vi "Output_Trav_Pos_low.vi"(4 "Positions to Output":T1) -> (1 "error out":errorcluster)   [LabVIEW 2011]
uses:
  Controls/Positions.ctl
  Globals/Trav_pos_global.vi
  <userlib>/LV-Link3/PolySubVIs/DtCreateAoutChan.vi
  Route mapping/Route_mapping_global.vi
  <userlib>/LV-Link3/PolySubVIs/DtOLWriteSingle.vi
  <userlib>/LV-Link3/PolySubVIs/DtOLWriteMultiple2D.vi
panel:
  out "X, Y, Z":dbl[](array[numeric])
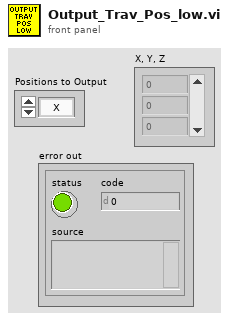
[diagram p1: front panel]
types:
  T1 = typedef "Positions.ctl" = enum16{"X", "Y", "Z", "XY", "XZ", "YZ", "XYZ"}
  T2 = typedef "Box_size.ctl" = cluster{"Max":dbl, "Min":dbl}[]
  T3 = enum32{"Bad", "Idle", "Run top level", "Running"}
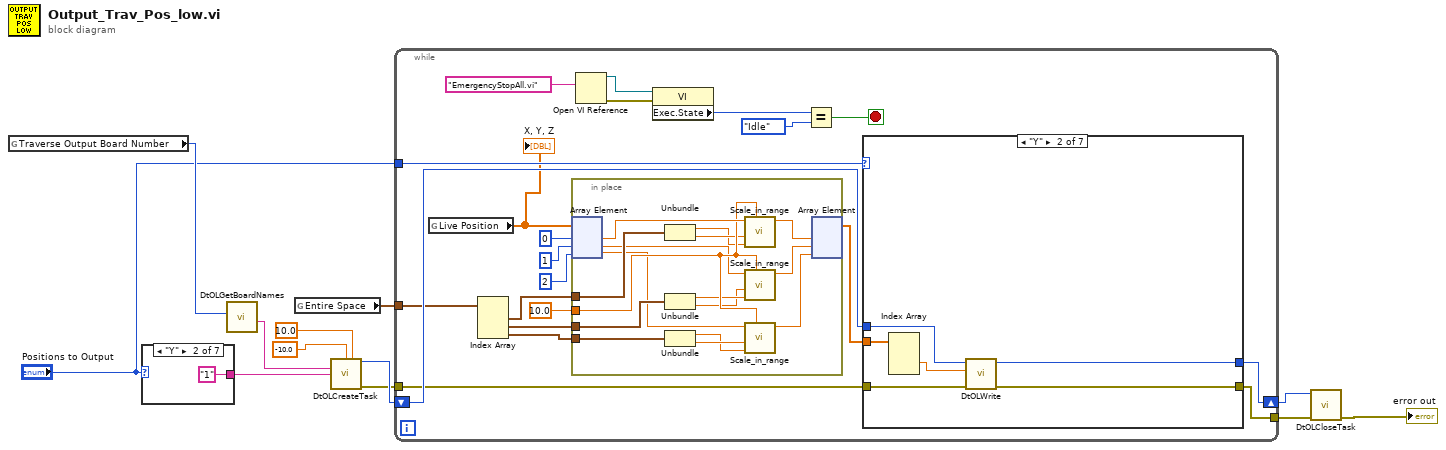
[diagram p0: block diagram]
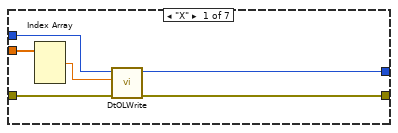
[diagram p2: hidden frame]
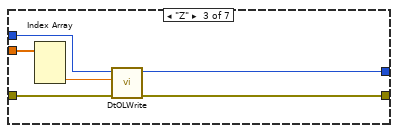
[diagram p3: hidden frame]
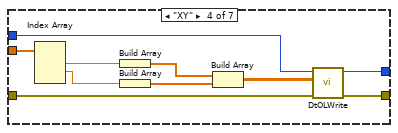
[diagram p4: hidden frame]
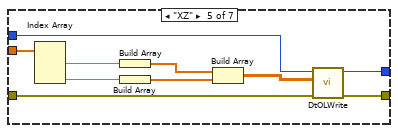
[diagram p5: hidden frame]
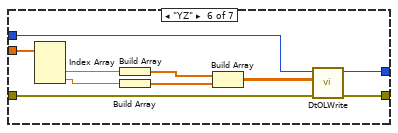
[diagram p6: hidden frame]
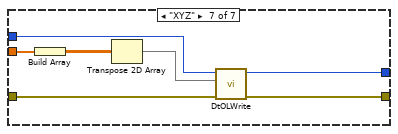
[diagram p7: hidden frame]
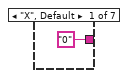
[diagram p8: hidden frame]
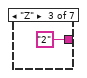
[diagram p9: hidden frame]
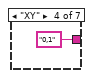
[diagram p10: hidden frame]
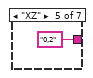
[diagram p11: hidden frame]
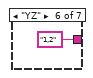
[diagram p12: hidden frame]
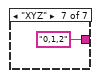
[diagram p13: hidden frame]
diagram:
  n1 = global read "Trav_pos_global.vi" "Traverse Output Board Number"() -> (w6:u32)
  n2 = case shown="\"Y\"" "Positions to Output" {
    tunnel: ["0" ("Channel") "1" ("Channel") "2" ("Channel") "0,1" ("Channel") "0,2" ("Channel") "1,2" ("Channel") "0,1,2" ("Channel")] -> w8
    frame "X", Default {
    }
    frame "Y" {
    }
    frame "Z" {
    }
    frame "XY" {
    }
    frame "XZ" {
    }
    frame "YZ" {
    }
    frame "XYZ" {
    }
  }
  n3 = call <userlib>:"DtOLGetBoardNames.vi"("Select Board"=w6) -> ("Board Name"=w9:string)  [unwired: 8 in, 2 out]
  n4 = global read "Route_mapping_global.vi" "Entire Space"() -> (w5:T2)
  n5 = call-poly <userlib>:"DtOLCreateTask.vi"("Range Min"=-10.0, "Range Max"=10.0, "Board Name"=w9, "Channel"=w8) -> ("Task out"=w10:i32, "error out"=w7:errorcluster)  [unwired: 9 in, 1 out]
  n6 = while {
    shift-right: [w40] -> w1
    shift-left: w10 -> [w39]
    tunnel: "Positions to Output" -> [w38]
    tunnel: w7 -> [w31]
    tunnel: [w30] -> w3
    tunnel: w5 -> [w27]
    stop <- w32 stop-if-true
    n7 = global read "Trav_pos_global.vi" "Live Position"() -> (w20:dbl[])
    "X, Y, Z" <- w20
    n8 = Index Array(array=w27) -> (element #1=w26:cluster{"Max":dbl, "Min":dbl}, element #2=w25:cluster{"Max":dbl, "Min":dbl}, element #3=w24:cluster{"Max":dbl, "Min":dbl})  [unwired: 3 in]
    n9 = in-place {
      in-place-border: 10.0 ("Scale Factor") -> [w55]
      in-place-border: w26 -> [w54]
      in-place-border: w25 -> [w51]
      in-place-border: w24 -> [w50]
      n10 = in-place-array #1(w20, 0, 1, 2) -> (w56:dbl, w45:dbl, w44:dbl)
      n11 = Unbundle(w54) -> ("Max"=w52:dbl, "Min"=w53:dbl)
      n12 = Unbundle(w51) -> ("Max"=w47:dbl, "Min"=w46:dbl)
      n13 = Unbundle(w50) -> ("Max"=w48:dbl, "Min"=w49:dbl)
      n14 = call "Scale_in_range.vi"("Scale Factor"=w55, "Maximum Range"=w52, "Minimum Range"=w53, "x"=w56) -> ("Scaled x"=w43:dbl)  [unwired: 7 in]
      n15 = call "Scale_in_range.vi"("Scale Factor"=w55, "Maximum Range"=w47, "Minimum Range"=w46, "x"=w45) -> ("Scaled x"=w42:dbl)  [unwired: 7 in]
      n16 = call "Scale_in_range.vi"("Scale Factor"=w55, "Maximum Range"=w48, "Minimum Range"=w49, "x"=w44) -> ("Scaled x"=w41:dbl)  [unwired: 7 in]
      n17 = in-place-array #1(w43, w42, w41) -> (w29:dbl[])  [unwired: 3 out]
    }
    n18 = Open VI Reference(vi path="EmergencyStopAll.vi") -> (vi reference=w34:refnum<vi>, error out=w35:errorcluster)  [unwired: 5 in]
    n19 = property class="VI"(reference=w34, error in=w35) -> ("Exec.State"=w37:T3)  [unwired: 2 out]
    n20 = Equal?(x=w37, y=T3."Idle") -> (x = y?=w32:bool)
    n21 = case shown="\"Y\"" w38 {
      tunnel: [w62 w68 w74 w84 w94 w104 w109] -> w40
      tunnel: w39 -> [w61 w67 w73 w83 w93 w103 w110]
      tunnel: w29 -> [w59 w65 w72 w82 w92 w102 w111]
      tunnel: w31 -> [w58 w64 w70 w76 w86 w96 w106]
      tunnel: [w57 w63 w69 w75 w85 w95 w105] -> w30
      frame "X" {
        n22 = Index Array(array=w59) -> (element #1=w60:dbl)  [unwired: 3 in, 2 out]
        n23 = call-poly <userlib>:"DtOLWrite.vi"("error in (no error)"=w58, "Data In"=w60, "Task in"=w61) -> ("error out"=w57:errorcluster, "Task out"=w62:i32)  [unwired: 7 in]
      }
      frame "Y" {
        n24 = Index Array(array=w65) -> (element #2=w66:dbl)  [unwired: 3 in, 2 out]
        n25 = call-poly <userlib>:"DtOLWrite.vi"("error in (no error)"=w64, "Data In"=w66, "Task in"=w67) -> ("error out"=w63:errorcluster, "Task out"=w68:i32)  [unwired: 7 in]
      }
      frame "Z" {
        n26 = Index Array(array=w72) -> (element #3=w71:dbl)  [unwired: 3 in, 2 out]
        n27 = call-poly <userlib>:"DtOLWrite.vi"("error in (no error)"=w70, "Data In"=w71, "Task in"=w73) -> ("error out"=w69:errorcluster, "Task out"=w74:i32)  [unwired: 7 in]
      }
      frame "XY" {
        n28 = Index Array(array=w82) -> (element #1=w81:dbl, element #2=w80:dbl)  [unwired: 3 in, 1 out]
        n29 = Build Array(w81) -> (w78:dbl[])
        n30 = Build Array(w80) -> (w79:dbl[])
        n31 = Build Array(w78, w79) -> (w77:dbl[][])
        n32 = call-poly <userlib>:"DtOLWrite.vi"("error in (no error)"=w76, "Data in"=w77, "Task in"=w83) -> ("error out"=w75:errorcluster, "Task out"=w84:i32)  [unwired: 6 in, 1 out]
      }
      frame "XZ" {
        n33 = Index Array(array=w92) -> (element #1=w91:dbl, element #3=w87:dbl)  [unwired: 3 in, 1 out]
        n34 = Build Array(w91) -> (w89:dbl[])
        n35 = Build Array(w87) -> (w90:dbl[])
        n36 = Build Array(w89, w90) -> (w88:dbl[][])
        n37 = call-poly <userlib>:"DtOLWrite.vi"("error in (no error)"=w86, "Data in"=w88, "Task in"=w93) -> ("error out"=w85:errorcluster, "Task out"=w94:i32)  [unwired: 6 in, 1 out]
      }
      frame "YZ" {
        n38 = Index Array(array=w102) -> (element #2=w97:dbl, element #3=w98:dbl)  [unwired: 3 in, 1 out]
        n39 = Build Array(w97) -> (w100:dbl[])
        n40 = Build Array(w98) -> (w101:dbl[])
        n41 = Build Array(w100, w101) -> (w99:dbl[][])
        n42 = call-poly <userlib>:"DtOLWrite.vi"("error in (no error)"=w96, "Data in"=w99, "Task in"=w103) -> ("error out"=w95:errorcluster, "Task out"=w104:i32)  [unwired: 6 in, 1 out]
      }
      frame "XYZ" {
        n43 = Build Array(w111) -> (w108:dbl[][])
        n44 = Transpose 2D Array(2D array=w108) -> (transposed array=w107:dbl[][])
        n45 = call-poly <userlib>:"DtOLWrite.vi"("error in (no error)"=w106, "Data in"=w107, "Task in"=w110) -> ("error out"=w105:errorcluster, "Task out"=w109:i32)  [unwired: 6 in, 1 out]
      }
    }
  }
  n46 = call <userlib>:"DtOLCloseTask.vi"("Error in"=w3, "Task in"=w1) -> ("Error Out"=→"error out":errorcluster)  [unwired: 9 in]
